vi "Derivative action.vi"(1 "iteration":i32, 2 "dt":dbl format="%.2f", 3 "process variable":dbl format="%.2f", 4 "Kd":dbl format="%.4f") -> (0 "derivative action":dbl format="%.2f")   [LabVIEW 2017, in "NI_PID__prctrl compat.lvlib"]
doc: "This function calculates the derivative action of the PID controller on the process variable."
uses:
  <vilib>/addons/control/pid/NI_PID__prctrl compat.lvlib
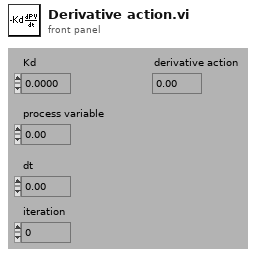
[diagram p1: front panel]
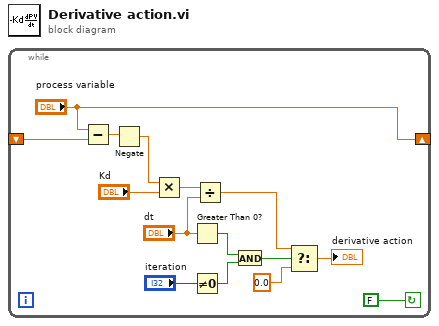
[diagram p0: block diagram]
diagram:
  n1 = while {
    shift-left: _ -> [w2]
    shift-right: ["process variable"] -> _
    stop <- FALSE continue-if-true
    n2 = Subtract(x="process variable", y=w2) -> (x-y=w13:dbl)
    n3 = Negate(x=w13) -> (-x=w14:dbl)
    n4 = Multiply(x=w14, y="Kd") -> (x*y=w5:dbl)
    n5 = Greater Than 0?(x="dt") -> (x > 0?=w8:bool)
    n6 = Not Equal To 0?(x="iteration") -> (x != 0?=w9:bool)
    n7 = Divide(x=w5, y="dt") -> (x/y=w6:dbl)
    n8 = And(x=w8, y=w9) -> (x .and. y?=w10:bool)
    n9 = Select(t=w6, s=w10, f=0.0) -> (s? t:f=→"derivative action":dbl)
  }
